vi "SE FP behavior point to dock.vi"(1 "GPS":cluster{"X pos":i32, "Y pos":i32, "Heading":dbl}={"X pos"=250, "Y pos"=430, "Heading"=180.0}, 2 "IR Sensors":T2(array[cluster]), 3 "GPS Initial":cluster{"X pos":i32, "Y pos":i32, "Heading":dbl}={"X pos"=-1, "Y pos"=-1, "Heading"=-1.0}, 4 "Behavior\nVelocity":dbl, 5 "Activate?":bool=TRUE, 6 "Camera Data":T1) -> (0 "Dock Array":dbl[](array[numeric]))   [LabVIEW 2014]
uses:
  <vilib>/addons/control/pid/pid.llb/PID (DBL).vi
  <vilib>/addons/control/pid/NI_PID_pid.lvlib
panel:
  out "Waveform Graph":cluster{dbl, dbl, dbl[]}(graph)
  # "Dock"
  # "Current"
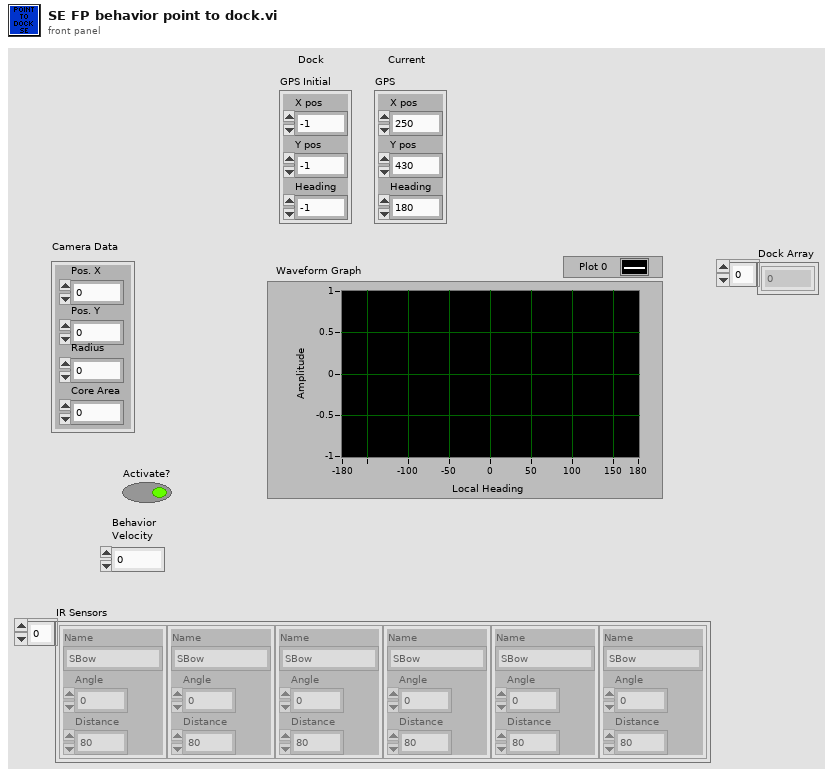
[diagram p1: front panel]
types:
  T1 = cluster{"Pos. X":i32, "Pos. Y":i32, "Radius":i32, "Core Area":i32}
  T2 = cluster{"Name":string, "Angle":dbl, "Distance":dbl}[]
  T3 = cluster{"Name":string, "Angle":dbl, "Distance":dbl}
  T4 = cluster{"proportional gain (Kc)":dbl, "integral time (Ti, min)":dbl, "derivative time (Td, min)":dbl}
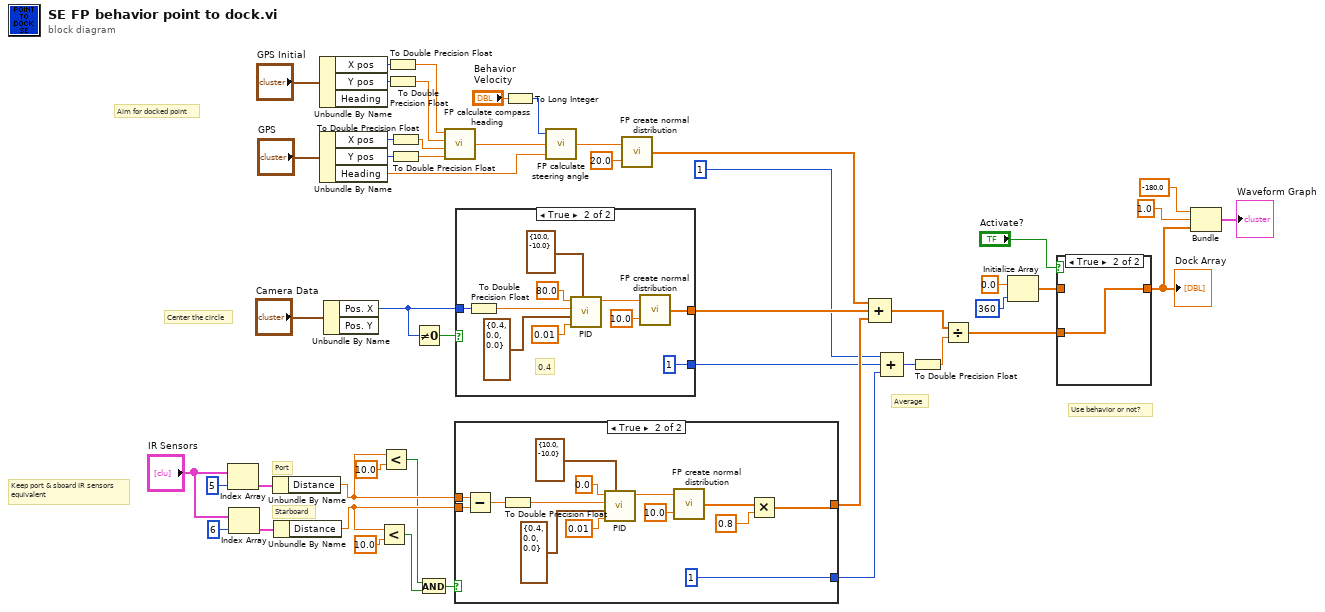
[diagram p0: block diagram]
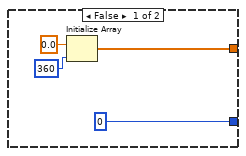
[diagram p2: hidden frame]
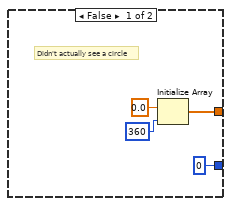
[diagram p3: hidden frame]
diagram:
  # "Use behavior or not?"
  # "Average"
  # "Keep port & sboard IR sensors\nequivalent"
  # "Starboard"
  # "Port"
  # "Center the circle"
  # "Aim for docked point"
  n1 = Index Array(array="IR Sensors", index=5) -> (element=w44:T3)
  n2 = Index Array(array="IR Sensors", index=6) -> (element=w20:T3)
  n3 = Unbundle By Name(w44) -> ("Distance"=w17:dbl)
  n4 = Unbundle By Name(w20) -> ("Distance"=w14:dbl)
  n5 = Unbundle By Name("GPS Initial") -> ("X pos"=w37:i32, "Y pos"=w36:i32)  [unwired: 1 out]
  n6 = Unbundle By Name("GPS") -> ("X pos"=w41:i32, "Y pos"=w40:i32, "Heading"=w29:dbl)
  n7 = Unbundle By Name("Camera Data") -> ("Pos. X"=w22:i32)  [unwired: 1 out]
  n8 = Less?(x=w14, y=10.0) -> (x < y?=w11:bool)
  n9 = Less?(x=w17, y=10.0) -> (x < y?=w12:bool)
  n10 = To Double Precision Float(number=w37) -> (double precision float=w35:dbl)
  n11 = To Double Precision Float(number=w36) -> (double precision float=w34:dbl)
  n12 = To Double Precision Float(number=w41) -> (double precision float=w39:dbl)
  n13 = To Double Precision Float(number=w40) -> (double precision float=w38:dbl)
  n14 = Not Equal To 0?(x=w22) -> (x != 0?=w21:bool)
  n15 = And(x=w12, y=w11) -> (x .and. y?=w13:bool)
  n16 = call "FP calculate compass heading.vi"("Y Location"=w38, "X Location"=w39, "Waypoint Y"=w34, "Waypoint X"=w35) -> ("Heading"=w31:dbl)
  n17 = case shown="True" w13 {
    tunnel: w14 -> [_ w62]
    tunnel: w17 -> [_ w58]
    tunnel: [w51 w55] -> w8
    tunnel: [0 1] -> w5
    frame False {
      n18 = Initialize Array(0.0 ("element"), 360 ("dimension size")) -> (w51:dbl[])
    }
    frame True {
      n19 = Subtract(x=w58, y=w62) -> (x-y=w61:dbl)
      n20 = To Double Precision Float(number=w61) -> (double precision float=w65:dbl)
      n21 = call-poly <vilib>:"PID.vi"("output range"=cluster{"output high":dbl, "output low":dbl} {"output high"=10.0, "output low"=-10.0}, "dt (s)"=0.01, "PID gains"=T4 {"proportional gain (Kc)"=0.4, "integral time (Ti, min)"=0.0, "derivative time (Td, min)"=0.0}, "process variable"=w65, "setpoint"=0.0) -> ("output"=w66:dbl)  [unwired: 5 in, 1 out]
      n22 = call "FP create normal distribution.vi"("std (Normal)"=10.0, "mean"=w66) -> ("ACT array"=w56:dbl[])
      n23 = Multiply(x=w56, y=0.8) -> (x*y=w55:dbl[])
    }
  }
  n24 = case shown="True" w21 {
    tunnel: w22 -> [_ w74]
    tunnel: [w69 w73] -> w9
    tunnel: [0 1] -> w6
    frame False {
      # "Didn't actually see a circle"
      n25 = Initialize Array(0.0 ("element"), 360 ("dimension size")) -> (w69:dbl[])
    }
    frame True {
      # "0.4"
      n26 = To Double Precision Float(number=w74) -> (double precision float=w77:dbl)
      n27 = call-poly <vilib>:"PID.vi"("output range"=cluster{"output high":dbl, "output low":dbl} {"output high"=10.0, "output low"=-10.0}, "dt (s)"=0.01, "PID gains"=T4 {"proportional gain (Kc)"=0.4, "integral time (Ti, min)"=0.0, "derivative time (Td, min)"=0.0}, "process variable"=w77, "setpoint"=80.0) -> ("output"=w76:dbl)  [unwired: 5 in, 1 out]
      n28 = call "FP create normal distribution.vi"("std (Normal)"=10.0, "mean"=w76) -> ("ACT array"=w73:dbl[])
    }
  }
  n29 = To Long Integer(number="Behavior\nVelocity") -> (32bit integer=w28:i32)
  n30 = call "FP calculate steering angle.vi"("Compass\nheading"=w29, "New heading"=w31, "Speed"=w28) -> ("Local Steering Angle"=w30:dbl)
  n31 = call "FP create normal distribution.vi"("std (Normal)"=20.0, "mean"=w30) -> ("ACT array"=w10:dbl[])
  n32 = Compound Arithmetic op=ADD(w10, w9, w8) -> (w4:dbl[])
  n33 = Compound Arithmetic op=ADD(1, w6, w5) -> (w3:i32)
  n34 = To Double Precision Float(number=w3) -> (double precision float=w2:dbl)
  n35 = Divide(x=w4, y=w2) -> (x/y=w1:dbl[])
  n36 = Initialize Array(0.0 ("element"), 360 ("dimension size")) -> (w25:dbl[])
  n37 = case shown="True" "Activate?" {
    tunnel: w25 -> [w82 _]
    tunnel: [w82 w83] -> w24
    tunnel: w1 -> [_ w83]
    frame False {
    }
    frame True {
    }
  }
  "Dock Array" <- w24
  n38 = Bundle(-180.0, 1.0, w24) -> (→"Waveform Graph":cluster{dbl, dbl, dbl[]})  [unwired: 1 in]
